vi "Fc_MenuSelections.vi"(6 "Cluster References":T2, 7 "ItemTag":string, 8 "error in (no error)":errorcluster, 9 "Cluster in":T1, 10 "VI caller":refnum<vi>, 11 "WaveformGraph in":refnum<vi>) -> (0 "error out":errorcluster, 3 "Cluster out":T1)   [LabVIEW 2022 SP3]
doc: "This function is used to select possible selection in the current window plot."
uses:
  <vilib>/Analysis/1siggen.llb/Ramp Pattern by Samples.vi
  <vilib>/Analysis/NI_AALBase.lvlib
  <vilib>/gmath/NI_Gmath.lvlib
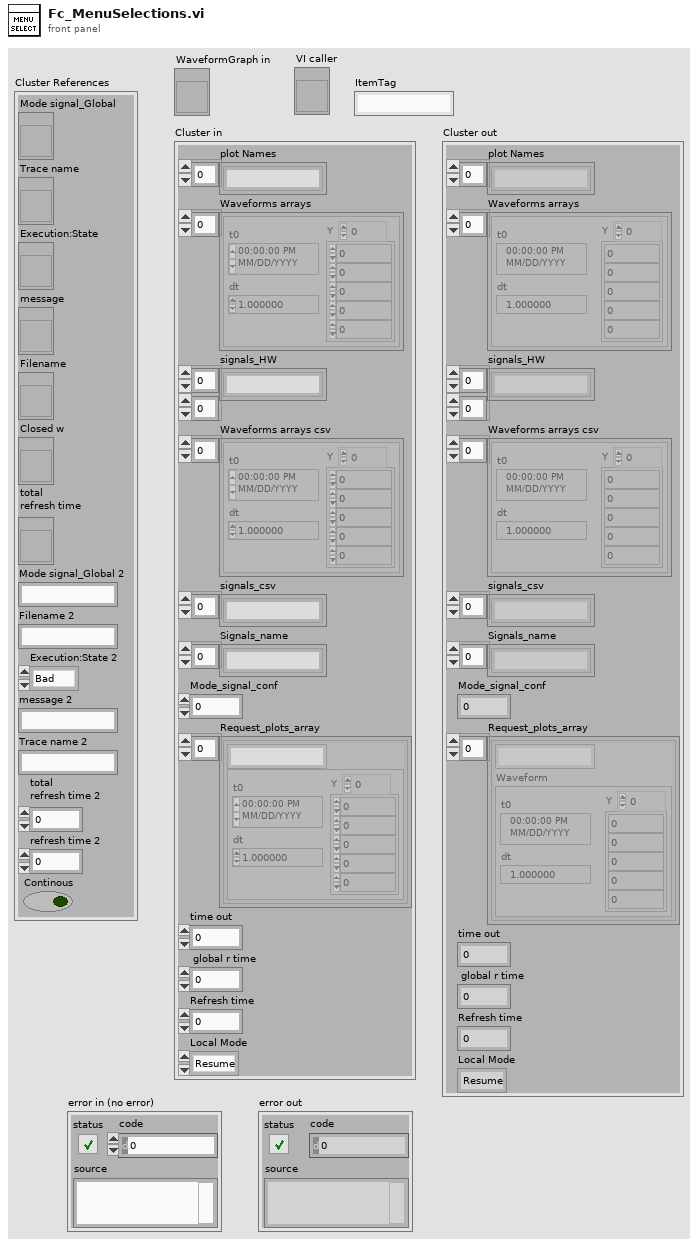
[diagram p1: front panel]
types:
  T1 = cluster{"plot Names":string[], "Waveforms arrays":waveform(dbl)[], "signals_HW":string[][], "Waveforms arrays csv":waveform(dbl)[], "signals_csv":string[], "Signals_name":string[], "Mode_signal_conf":u8, "Request_plots_array":cluster{string, "Waveform":waveform(dbl)}[], "time out":i32, " global r time":u32, "Refresh time":u32, "Local Mode":enum32{"Resume", "Hold"}}
  T2 = cluster{"Mode signal_Global":refnum<vi>, "Trace name":refnum<vi>, "Execution:State":refnum<vi>, "message":refnum<vi>, "Filename":refnum<vi>, "Closed w":refnum<vi>, "total \nrefresh time":refnum<vi>, "Mode signal_Global 2":string, "Filename 2":string, "Execution:State 2":enum32{"Bad", "Idle", "Run top level", "Running"}, "message 2":string, "Trace name 2":string, "total \nrefresh time 2":i32, "refresh time 2":i32, "Continous":bool}
  T3 = enum32{"Bad", "Idle", "Run top level", "Running"}
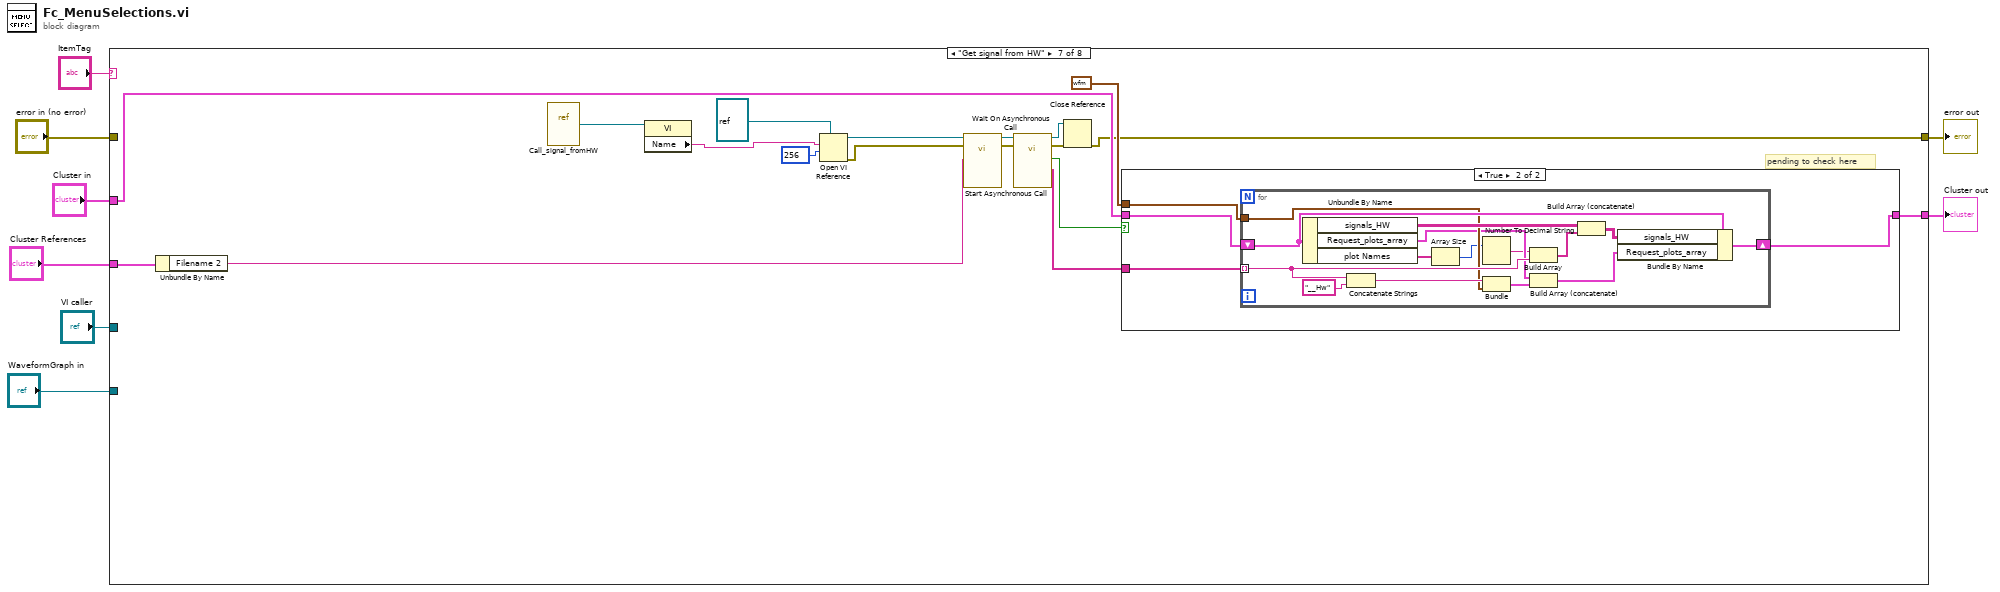
[diagram p0: block diagram]
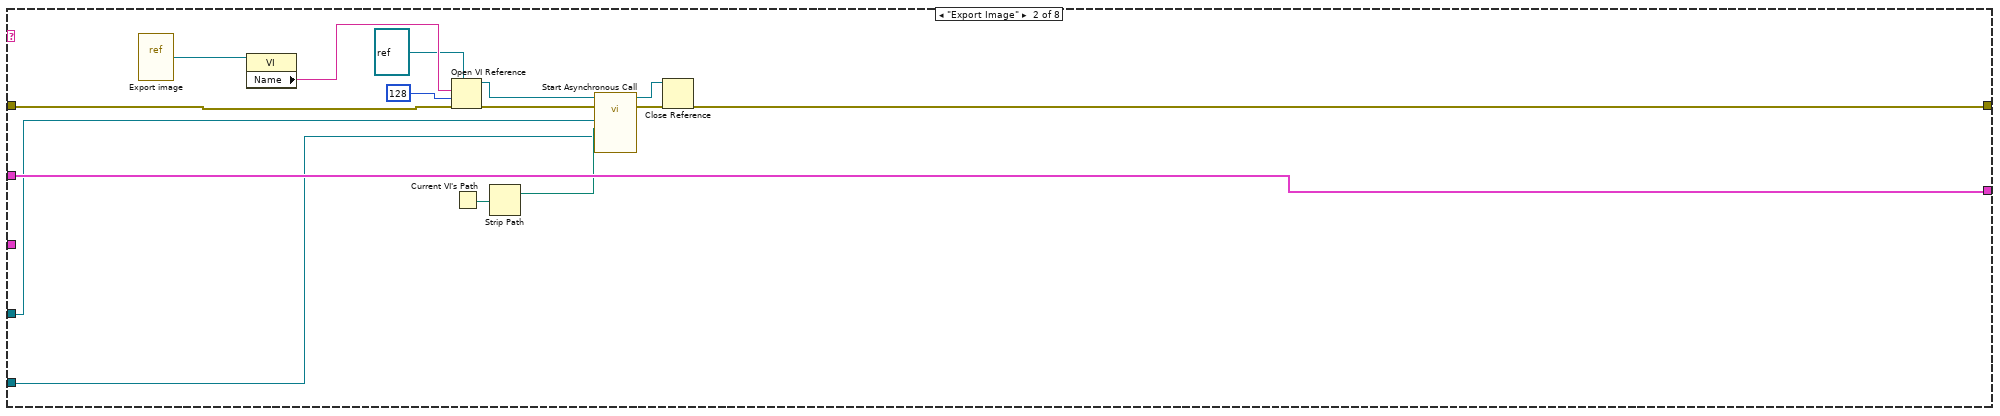
[diagram p3: hidden frame]
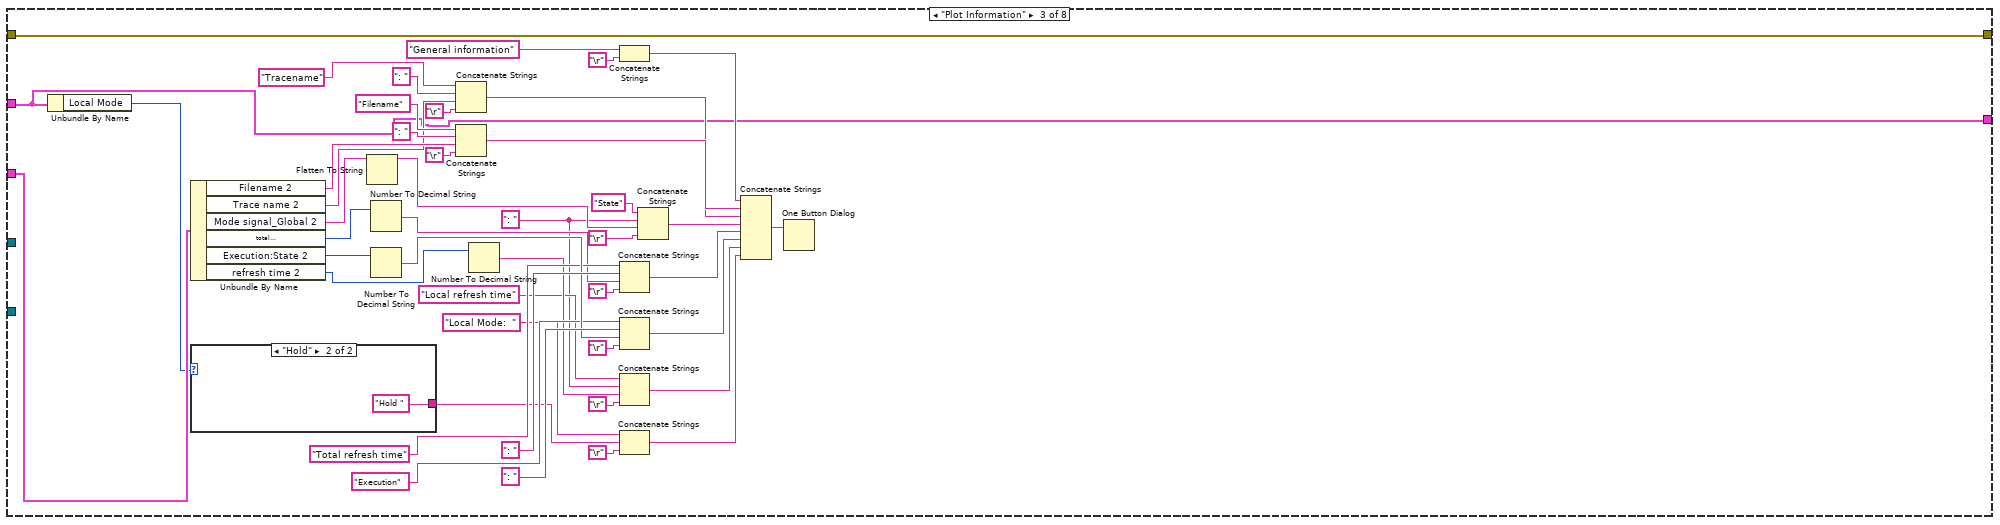
[diagram p4: hidden frame]
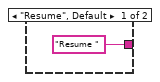
[diagram p5: hidden frame]
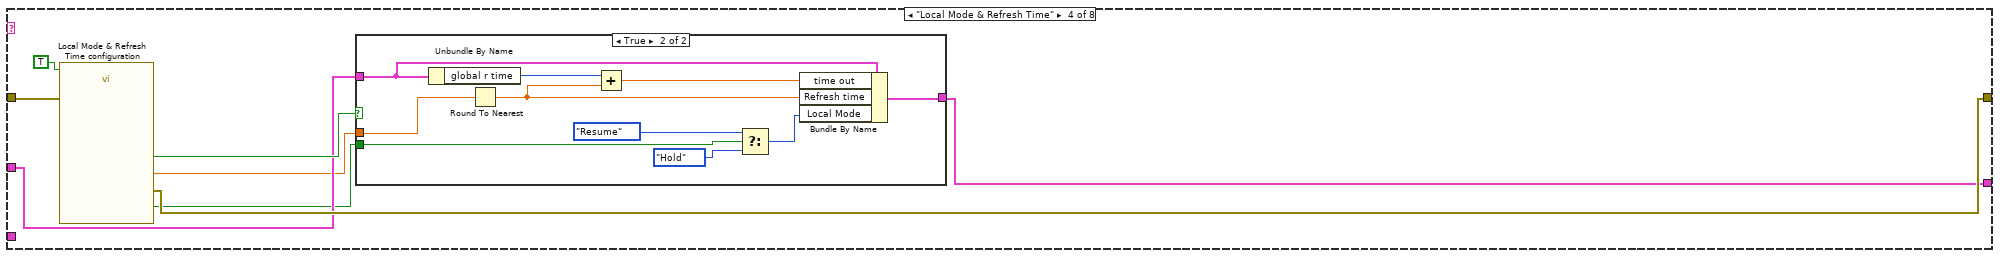
[diagram p6: hidden frame]
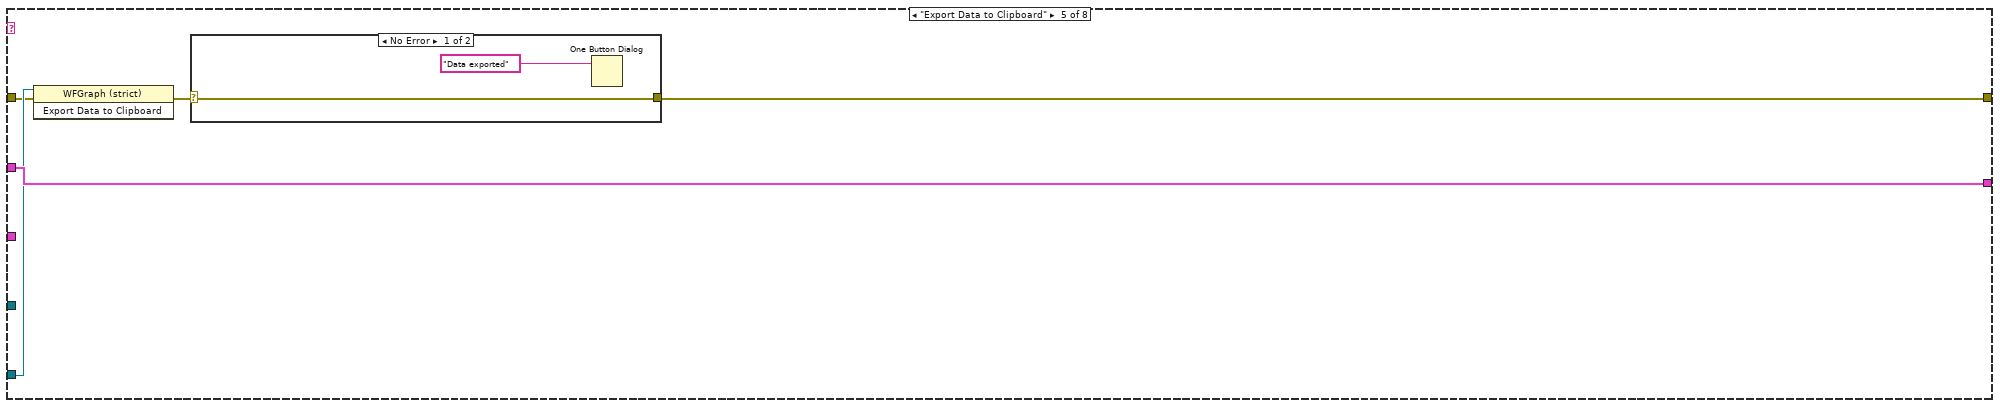
[diagram p8: hidden frame]
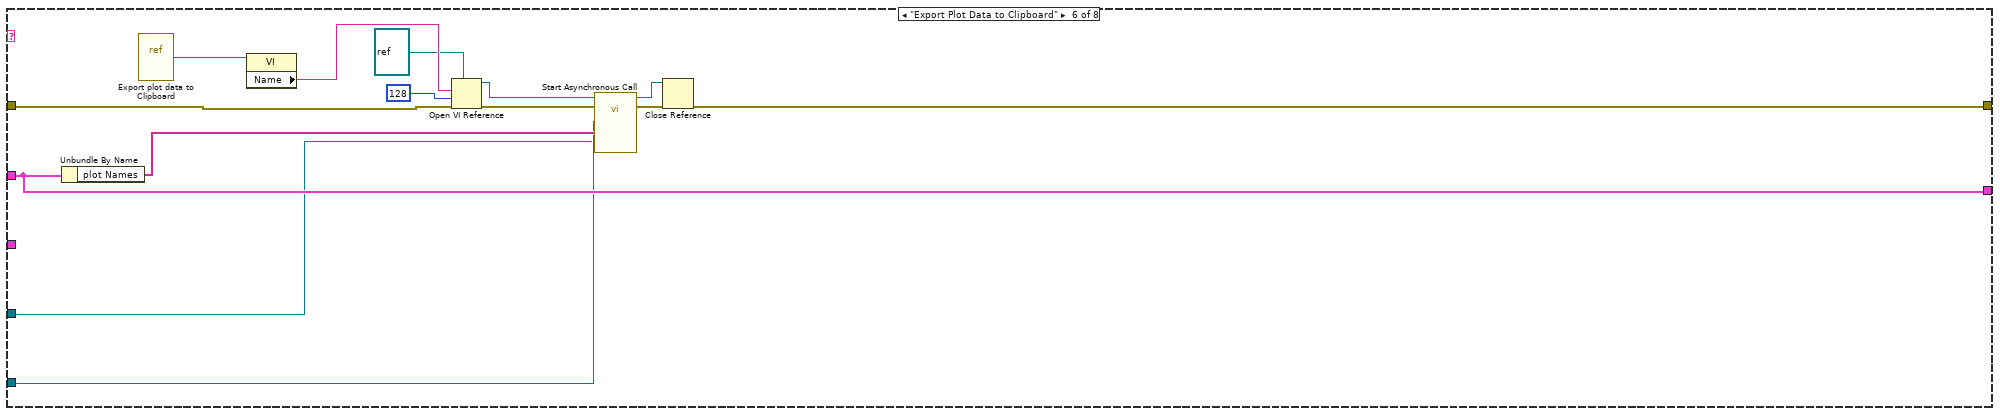
[diagram p10: hidden frame]
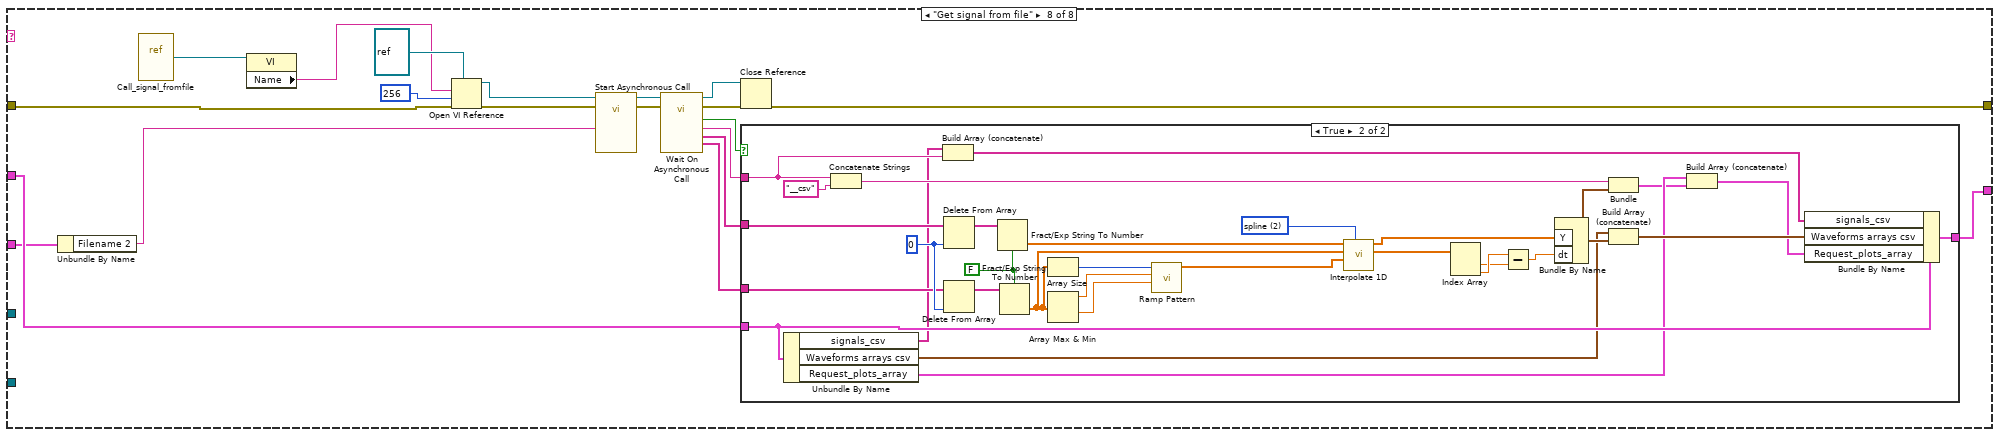
[diagram p12: hidden frame]
diagram:
  n1 = case shown="\"Get signal from HW\"" "ItemTag" {
    tunnel: [w10 w25 w31 w74 w96 w107 w127 w165] -> w4
    tunnel: "Cluster in" -> [w10 w25 w31 w76 w96 w107 w119 w166]
    tunnel: [w9 w14 w70 w78 w95 w103 w117 w155] -> w5
    tunnel: "error in (no error)" -> [w9 w13 w70 w79 w92 w102 _ w154]
    tunnel: "WaveformGraph in" -> [_ w12 _ _ w94 w101 _ _]
    tunnel: "VI caller" -> [_ w11 _ _ _ w100 _ _]
    tunnel: "Cluster References" -> [_ _ w69 _ _ _ w115 w153]
    frame "False", Default {
    }
    frame "Export Image" {
      n2 = vi-ref "Export image.vi"() -> (w19:refnum<vi>)
      n3 = property class="VI"(reference=w19) -> ("Name"=w21:string)  [unwired: 1 in, 2 out]
      n4 = Open VI Reference(type specifier VI Refnum (for type only)=refnum<vi> refnum ("reference"), vi path=w21, options=128, error in (no error)=w13) -> (vi reference=w22:refnum<vi>, error out=w23:errorcluster)  [unwired: 2 in]
      n5 = Current VI's Path() -> (path=w24:path)
      n6 = Strip Path(path=w24) -> (stripped path=w17:path)  [unwired: 1 out]
      n7 = call-by-ref "Start Asynchronous Call"(reference=w22, error in=w23, "Graph reference"=w12, "Folder selection"=w17, "VI caller"=w11) -> (reference out=w16:refnum<vi>, error out=w15:errorcluster)  [unwired: 8 in, 1 out]
      n8 = Close Reference(reference=w16, error in (no error)=w15) -> (error out=w14:errorcluster)
    }
    frame "Plot Information" {
      w33 = ": " ("string")
      n9 = Unbundle By Name(w31) -> ("Local Mode"=w30:enum32{"Resume", "Hold"})
      n10 = Unbundle By Name(w69) -> ("Filename 2"=w46:string, "Trace name 2"=w45:string, "Mode signal_Global 2"=w43:string, "total \nrefresh time 2"=w41:i32, "Execution:State 2"=w39:T3, "refresh time 2"=w35:i32)
      n11 = case shown="\"Hold\"" w30 {
        tunnel: ["Resume " ("string") "Hold " ("string")] -> w28
        frame "Resume", Default {
        }
        frame "Hold" {
        }
      }
      n12 = Flatten To String(anything=w43) -> (data string=w60:string)  [unwired: 3 in, 2 out]
      n13 = Number To Decimal String(number=w41) -> (decimal integer string=w40:string)  [unwired: 1 in]
      n14 = Number To Decimal String(number=w39) -> (decimal integer string=w53:string)  [unwired: 1 in]
      n15 = Concatenate Strings("Tracename" ("string"), ": " ("string"), w45, "\r") -> (w63:string)
      n16 = Concatenate Strings("Filename" ("string"), ": " ("string"), w46, "\r") -> (w64:string)
      n17 = Number To Decimal String(number=w35) -> (decimal integer string=w37:string)  [unwired: 1 in]
      n18 = Concatenate Strings("General information" ("string"), "\r") -> (w48:string)
      n19 = Concatenate Strings("Total refresh time" ("string"), ": " ("string"), w40, "\r") -> (w56:string)
      n20 = Concatenate Strings("Execution" ("string"), ": " ("string"), w53, "\r") -> (w52:string)
      n21 = Concatenate Strings("Local refresh time" ("Label.Text"), w33, w37, "\r") -> (w32:string)
      n22 = Concatenate Strings("Local Mode:  " ("string"), w28, "\r") -> (w26:string)
      n23 = Concatenate Strings("State" ("Label.Text"), w33, w60, "\r") -> (w59:string)
      n24 = Concatenate Strings(w48, w64, w63, w59, w56, w52, w32, w26) -> (w51:string)
      n25 = One Button Dialog(message=w51) -> ()  [unwired: 1 in, 1 out]
    }
    frame "Local Mode & Refresh Time" {
      n26 = call "Local Mode & Refresh Time configuration"("Enable"=TRUE, "error in (no error)"=w79) -> ("Refresh time"=w75:dbl, "Resume getting data"=w73:bool, "OK"=w77:bool, "error out"=w78:errorcluster)  [unwired: 14 in]
      n27 = case shown="True" w77 {
        tunnel: w76 -> [w81 w87]
        tunnel: w75 -> [_ w90]
        tunnel: [w81 w86] -> w74
        tunnel: w73 -> [_ w85]
        frame False {
        }
        frame True {
          n28 = Unbundle By Name(w87) -> ("global r time"=w91:u32)
          n29 = Round To Nearest(number=w90) -> (nearest integer value=w89:dbl)
          n30 = Add(x=w91, y=w89) -> (x+y=w88:dbl)
          n31 = Select(t=enum32{"Resume", "Hold"}."Resume" ("Local Mode"), s=w85, f=enum32{"Resume", "Hold"}."Hold" ("Local Mode")) -> (s? t:f=w82:enum32{"Resume", "Hold"})
          n32 = Bundle By Name(cluster=w87, "time out"=w88, "Refresh time"=w89, "Local Mode"=w82) -> (w86:T1)
        }
      }
    }
    frame "Export Data to Clipboard" {
      n33 = invoke class="WFGraph (strict)" method="Export Data to Clipboard"(reference=w94, error in=w92) -> (error out=w93:errorcluster)  [unwired: 1 in, 2 out]
      n34 = case shown="No Error" w93 {
        selector: w93 -> [w97 w99]
        tunnel: [w97 w99] -> w95
        frame No Error {
          n35 = One Button Dialog(message="Data exported") -> ()  [unwired: 1 in, 1 out]
        }
        frame Error {
        }
      }
    }
    frame "Export Plot Data to Clipboard" {
      n36 = Unbundle By Name(w107) -> ("plot Names"=w109:string[])
      n37 = vi-ref "Export plot data to Clipboard.vi"() -> (w104:refnum<vi>)
      n38 = property class="VI"(reference=w104) -> ("Name"=w113:string)  [unwired: 1 in, 2 out]
      n39 = Open VI Reference(type specifier VI Refnum (for type only)=refnum<vi> refnum ("reference"), vi path=w113, options=128, error in (no error)=w102) -> (vi reference=w112:refnum<vi>, error out=w111:errorcluster)  [unwired: 2 in]
      n40 = call-by-ref "Start Asynchronous Call"(reference=w112, error in=w111, "VI caller"=w100, "List Plots"=w109, "Graph reference"=w101) -> (reference out=w106:refnum<vi>, error out=w105:errorcluster)  [unwired: 2 in, 1 out]
      n41 = Close Reference(reference=w106, error in (no error)=w105) -> (error out=w103:errorcluster)
    }
    frame "Get signal from HW" {
      # "pending to check here"
      n42 = Unbundle By Name(w115) -> ("Filename 2"=w116:string)
      n43 = vi-ref "Call_signal_fromHW.vi"() -> (w128:refnum<vi>)
      n44 = property class="VI"(reference=w128) -> ("Name"=w120:string)  [unwired: 1 in, 2 out]
      n45 = Open VI Reference(type specifier VI Refnum (for type only)=refnum<vi> refnum ("reference"), vi path=w120, options=256) -> (vi reference=w129:refnum<vi>, error out=w131:errorcluster)  [unwired: 3 in]
      n46 = call-by-ref "Start Asynchronous Call"(reference=w129, error in=w131, "Plot window"=w116) -> (reference out=w125:refnum<vi>, error out=w126:errorcluster)  [unwired: 3 in, 2 out]
      n47 = call-by-ref "Wait On Asynchronous Call"(reference=w125, error in=w126) -> (reference out=w124:refnum<vi>, error out=w123:errorcluster, "Selected signals"=w114:string[], "Ready?"=w122:bool)  [unwired: 4 in]
      n48 = Close Reference(reference=w124, error in (no error)=w123) -> (error out=w117:errorcluster)
      n49 = case shown="True" w122 {
        tunnel: w114 -> [_ w136]
        tunnel: [w132 w134] -> w127
        tunnel: w119 -> [w132 w135]
        tunnel: waveform(dbl) {"t0"=timestamp(0 s since 1904-01-01), "dt"=1.0, "Y"=[]} ("Waveform") -> [_ w133]
        frame False {
        }
        frame True {
          n50 = for {
            tunnel: w136 -> [w150] mode=indexing
            tunnel: w133 -> [w143]
            shift-right: [w145] -> w134
            shift-left: w135 -> [w149]
            n51 = Unbundle By Name(w149) -> ("signals_HW"=w148:string[][], "Request_plots_array"=w142:cluster{string, "Waveform":waveform(dbl)}[], "plot Names"=w139:string[])
            n52 = Concatenate Strings(w150, "__Hw" ("string")) -> (w144:string)
            n53 = Array Size(array=w139) -> (size(s)=w138:i32)
            n54 = Number To Decimal String(number=w138) -> (decimal integer string=w137:string)  [unwired: 1 in]
            n55 = Bundle(w144, "Waveform"=w143) -> (w141:cluster{string, "Waveform":waveform(dbl)})  [unwired: 1 in]
            n56 = Build Array(w137, w150) -> (w147:string[])
            n57 = Build Array (concatenate)(w142, w141) -> (w140:cluster{string, "Waveform":waveform(dbl)}[])
            n58 = Build Array (concatenate)(w148, w147) -> (w146:string[][])
            n59 = Bundle By Name(cluster=w149, "signals_HW"=w146, "Request_plots_array"=w140) -> (w145:T1)
          }
        }
      }
    }
    frame "Get signal from file" {
      n60 = Unbundle By Name(w153) -> ("Filename 2"=w152:string)
      n61 = vi-ref "Call_signal_fromfile.vi"() -> (w169:refnum<vi>)
      n62 = property class="VI"(reference=w169) -> ("Name"=w163:string)  [unwired: 1 in, 2 out]
      n63 = Open VI Reference(type specifier VI Refnum (for type only)=refnum<vi> refnum, vi path=w163, options=256, error in (no error)=w154) -> (vi reference=w167:refnum<vi>, error out=w171:errorcluster)  [unwired: 2 in]
      n64 = call-by-ref "Start Asynchronous Call"(reference=w167, error in=w171, "Plot window"=w152) -> (reference out=w164:refnum<vi>, error out=w162:errorcluster)  [unwired: 3 in, 4 out]
      n65 = call-by-ref "Wait On Asynchronous Call"(reference=w164, error in=w162) -> (reference out=w157:refnum<vi>, error out=w156:errorcluster, "Y subarray"=w158:string[], "X subarray"=w159:string[], "Curve name"=w160:string, "Ready?"=w161:bool)  [unwired: 4 in]
      n66 = Close Reference(reference=w157, error in (no error)=w156) -> (error out=w155:errorcluster)
      n67 = case shown="True" w161 {
        tunnel: w159 -> [_ w202]
        tunnel: w158 -> [_ w201]
        tunnel: w160 -> [_ w184]
        tunnel: w166 -> [w172 w178]
        tunnel: [w172 w179] -> w165
        frame False {
        }
        frame True {
          w193 = 2 items=["nearest", "linear", "spline", "cubic Hermite", "Lagrange"] ("method")
          w198 = FALSE ("use system decimal point (T)")
          w203 = 0 ("index")
          n68 = Unbundle By Name(w178) -> ("signals_csv"=w176:string[], "Waveforms arrays csv"=w177:waveform(dbl)[], "Request_plots_array"=w175:cluster{string, "Waveform":waveform(dbl)}[])
          n69 = Concatenate Strings(w184, "__csv" ("string")) -> (w183:string)
          n70 = Build Array (concatenate)(w176, w184) -> (w181:string[])
          n71 = Delete From Array(array=w202, index=w203) -> (array with subset deleted=w199:string[])  [unwired: 1 in, 1 out]
          n72 = Delete From Array(array=w201, index=w203) -> (array with subset deleted=w200:string[])  [unwired: 1 in, 1 out]
          n73 = Fract/Exp String To Number(use system decimal point (T)=w198, string=w199) -> (number=w190:dbl[])  [unwired: 2 in, 1 out]
          n74 = Fract/Exp String To Number(use system decimal point (T)=w198, string=w200) -> (number=w192:dbl[])  [unwired: 2 in, 1 out]
          n75 = Array Size(array=w192) -> (size(s)=w196:i32)
          n76 = Array Max & Min(array=w192) -> (max value=w195:dbl, min value=w194:dbl)  [unwired: 2 out]
          n77 = call-poly <vilib>:"Ramp Pattern.vi"("start"=w194, "end"=w195, "samples"=w196) -> ("Ramp Pattern"=w191:dbl[])  [unwired: 7 in, 1 out]
          n78 = call <vilib>:"Interpolate 1D.vi"("method"=w193, "xi"=w191, "X"=w192, "Y"=w190) -> ("xi used"=w189:dbl[], "yi"=w188:dbl[])  [unwired: 5 in, 1 out]
          n79 = Index Array(array=w189) -> (element #1=w186:dbl, element #2=w187:dbl)  [unwired: 2 in]
          n80 = Subtract(x=w187, y=w186) -> (x-y=w185:dbl)
          n81 = Bundle By Name("Y"=w188, "dt"=w185) -> (w182:waveform(dbl))  [unwired: 1 in]
          n82 = Bundle(w183, w182) -> (w174:cluster{string, waveform(dbl)})  [unwired: 1 in]
          n83 = Build Array (concatenate)(w177, w182) -> (w180:waveform(dbl)[])
          n84 = Build Array (concatenate)(w175, w174) -> (w173:cluster{string, "Waveform":waveform(dbl)}[])
          n85 = Bundle By Name(cluster=w178, "signals_csv"=w181, "Waveforms arrays csv"=w180, "Request_plots_array"=w173) -> (w179:T1)
        }
      }
    }
  }
  "error out" <- w5
  "Cluster out" <- w4
